vi "4.4.vi"() -> ()   [LabVIEW 2017]
panel:
  in  "温度计":dbl(slide) scale=-100.0..100.0
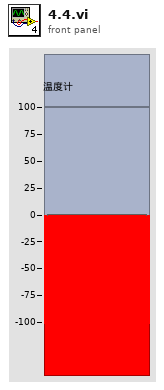
[diagram p1: front panel]
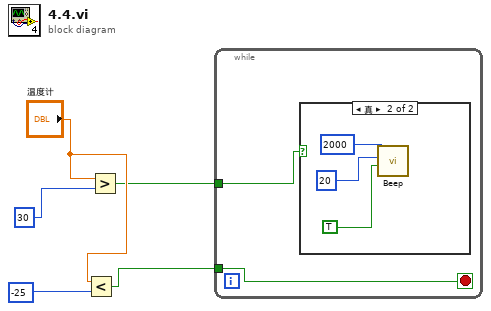
[diagram p0: block diagram]
diagram:
  n1 = Less?(x="温度计", y=-25) -> (x < y?=w2:bool)
  n2 = Greater?(x="温度计", y=30) -> (0:w1:bool)
  n3 = while {
    tunnel: w2 -> [w7]
    tunnel: w1 -> [w6]
    stop <- w7 stop-if-true
    n4 = case shown="真" w6 {
      frame False {
      }
      frame True {
        n5 = call <vilib>:"Beep.vi"("use system alert? (T)"=TRUE, "duration (msec)"=20, "frequency (Hz)"=2000) -> ()  [unwired: 9 in]
      }
    }
  }
